vi "Measurement Data Status.vi"(6 "Measurement Register Value To Set (0)":i32, 7 "Measurement Register To Set (0: Enable)":i32(ring) items=["Enable", "NTR", "PTR"], 8 "error in (no error)":errorcluster, 9 "Measurement Register To Check (0: Condition)":i32(ring) items=["Condition", "Enable", "Event", "NTR", "PTR"], 10 "Operation Mode (0: Check)":i32(ring) items=["Check", "Set"], 11 "VISA resource name":refnum<visa-resource-name>) -> (0 "error out":errorcluster, 2 "Measurement Register Status":bool[](array[boolean]), 3 "VISA resource name out":refnum<visa-resource-name>)   [LabVIEW 2020, in "Agilent B2900 Series.lvlib"]
doc: "Sets or checks the Measurement Data Status registers.\n\n<B>Note:</B> Use this VI only with other low-level VIs. The high-level VIs automatically incorporate this functionality. This VI does not check the instrument status."
uses:
  Agilent B2900 Series.lvlib
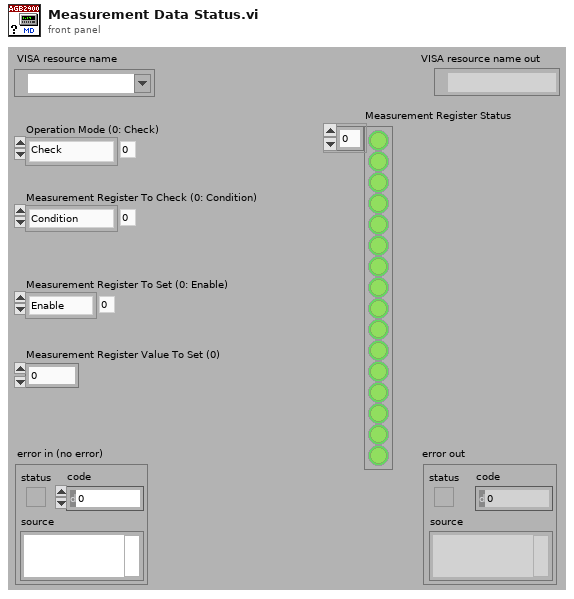
[diagram p1: front panel]
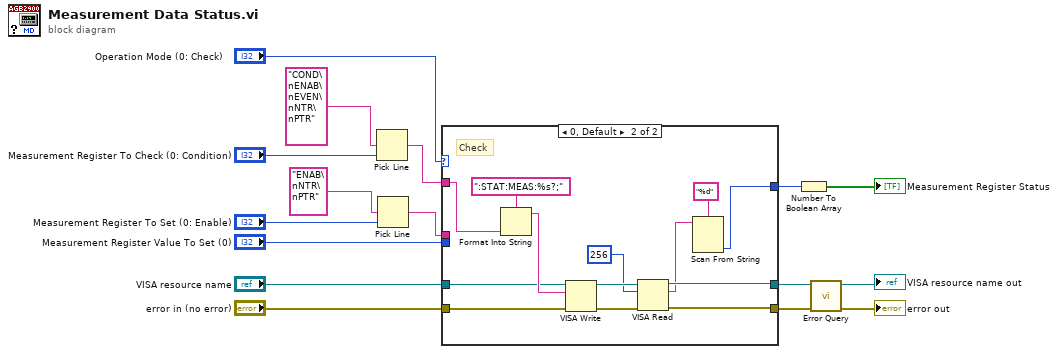
[diagram p0: block diagram]
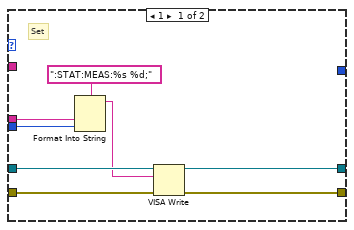
[diagram p2: hidden frame]
diagram:
  n1 = Pick Line(multi-line string="COND\nENAB\nEVEN\nNTR\nPTR", line index="Measurement Register To Check (0: Condition)") -> (output string=w11:string)  [unwired: 1 in]
  n2 = Pick Line(multi-line string="ENAB\nNTR\nPTR", line index="Measurement Register To Set (0: Enable)") -> (output string=w6:string)  [unwired: 1 in]
  n3 = case shown="0, Default" "Operation Mode (0: Check)" {
    tunnel: w11 -> [_ w36]
    tunnel: "VISA resource name" -> [w23 w34]
    tunnel: "error in (no error)" -> [w22 w33]
    tunnel: [w18 w30] -> w4
    tunnel: [w17 w29] -> w3
    tunnel: [_ w25] -> w8
    tunnel: w6 -> [w24 _]
    tunnel: "Measurement Register Value To Set (0)" -> [w19 _]
    frame 1 {
      # "Set"
      n4 = Format Into String(format string=":STAT:MEAS:%s %d;", w24, w19) -> (resulting string=w21:string)  [unwired: 2 in, 1 out]
      n5 = VISA Write(VISA resource name=w23, write buffer=w21, error in (no error)=w22) -> (VISA resource name out=w18:refnum<visa-resource-name>, error out=w17:errorcluster)  [unwired: 1 out]
    }
    frame 0, Default {
      # "Check"
      n6 = Format Into String(format string=":STAT:MEAS:%s?;", w36) -> (resulting string=w35:string)  [unwired: 2 in, 1 out]
      n7 = VISA Write(VISA resource name=w34, write buffer=w35, error in (no error)=w33) -> (VISA resource name out=w31:refnum<visa-resource-name>, error out=w32:errorcluster)  [unwired: 1 out]
      n8 = VISA Read(VISA resource name=w31, byte count=u32 256, error in (no error)=w32) -> (VISA resource name out=w30:refnum<visa-resource-name>, read buffer=w27:string, error out=w29:errorcluster)  [unwired: 1 out]
      n9 = Scan From String(format string="%d", input string=w27) -> (output 1=w25:i32)  [unwired: 3 in, 3 out]
    }
  }
  n10 = Number To Boolean Array(number=w8) -> (Boolean array=→"Measurement Register Status":bool[])
  n11 = call "Error Query.vi"("error in (no error)"=w3, "VISA resource name"=w4) -> ("error out"=→"error out":errorcluster, "VISA resource name out"=→"VISA resource name out":refnum<visa-resource-name>)  [unwired: 6 in, 2 out]
